vi "Close Input Test Connections.vi"(8 "error in":errorcluster, 10 "OPC UA server refnum":refnum<k21>, 11 "OPC UA runtime in":refnum<class "OPC UA Client runtime.lvclass">) -> (0 "error out":errorcluster)   [LabVIEW 2013, in "OPC UA Client Tests.lvlib"]
doc: "Close out OPC UA client's connection then stop and close the OPC UA server"
uses:
  OPC UA Client Tests.lvlib
  module/execution/OPC UA Client runtime.lvclass
  <vilib>/opcua/NI OPC UA Server.lvlib
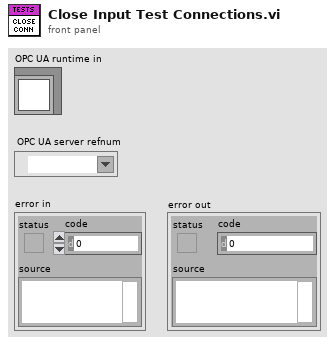
[diagram p1: front panel]
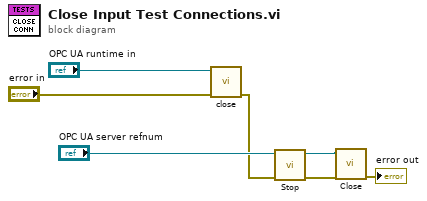
[diagram p0: block diagram]
diagram:
  n1 = call-dynamic <vilib>:"close.vi"("error in"="error in", "OPC UA runtime in"="OPC UA runtime in") -> ("error out"=w4:errorcluster)  [unwired: 9 in]
  n2 = call <vilib>:"Stop.vi"("error in (no error)"=w4, "OPC UA server refnum in"="OPC UA server refnum") -> ("error out"=w7:errorcluster, "OPC UA server refnum out"=w6:refnum<k21>)  [unwired: 8 in]
  n3 = call <vilib>:"Close.vi"("error in (no error)"=w7, "OPC UA server refnum in"=w6) -> ("error out"=→"error out":errorcluster)  [unwired: 9 in]
